vi "__replaceDupNames.vi"(10 "input names":string[](array[string])=["tt", "", "tt1", "tt0", "tt11", "", "Untitled1", "10t", "10t", "tt11", "Untitled", "tt001", "tt001", "tt2", "tt1.3", "tt1.3", "tt100", "tt100"]) -> (2 "output names":string[](array[string]))   [LabVIEW 2020]
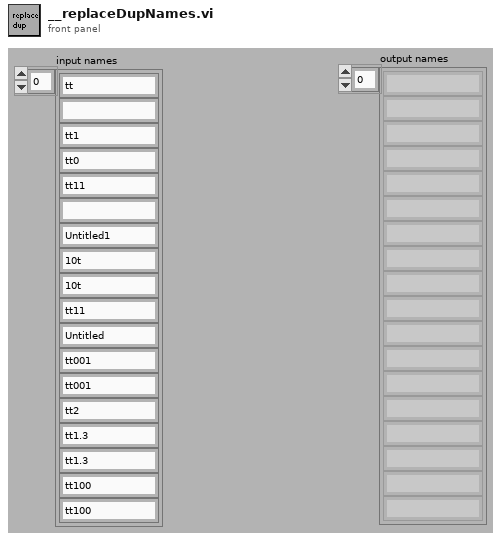
[diagram p1: front panel]
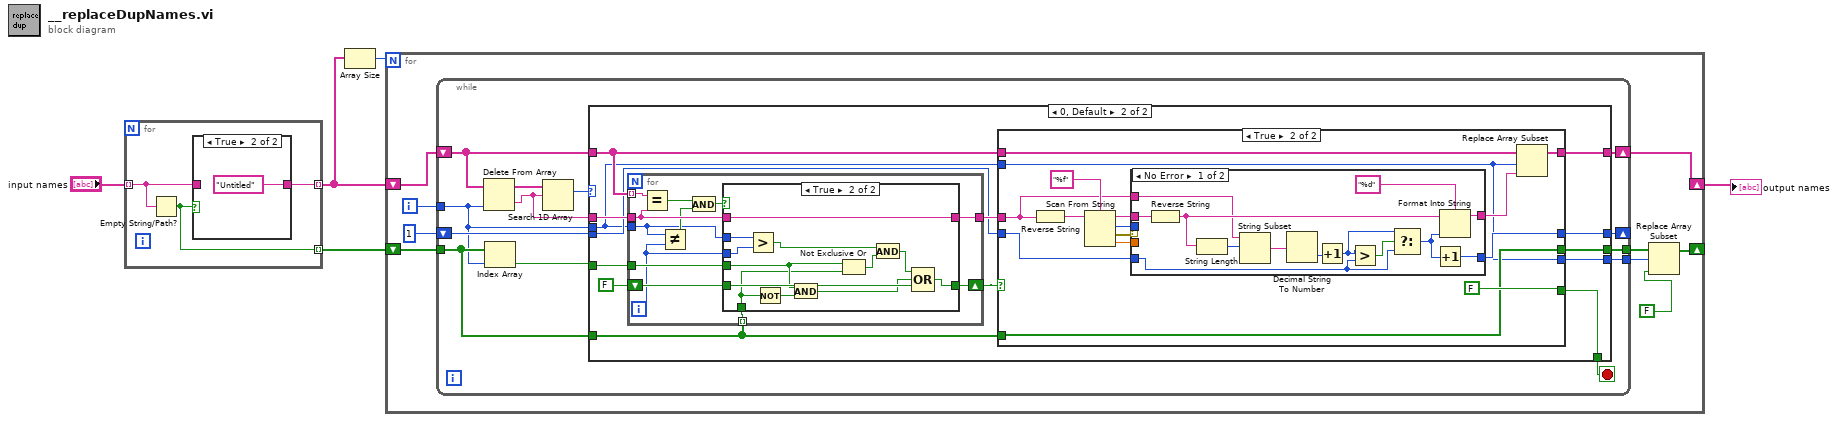
[diagram p0: block diagram]
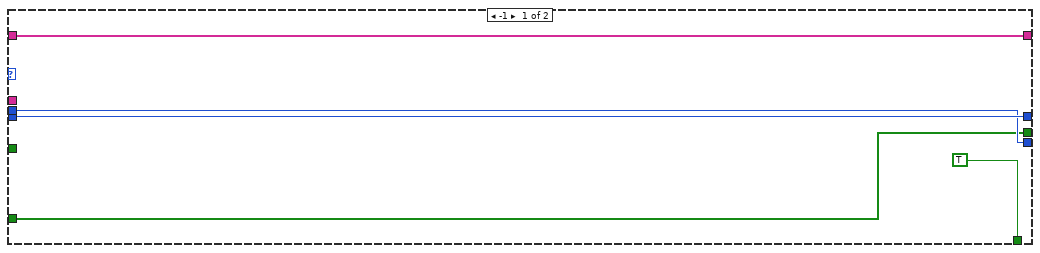
[diagram p2: hidden frame]
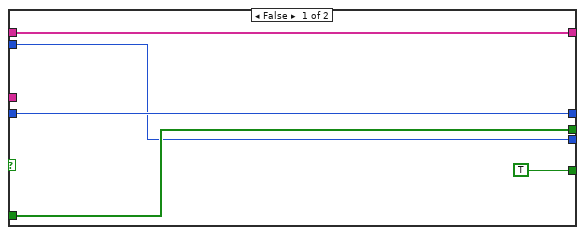
[diagram p4: hidden frame]
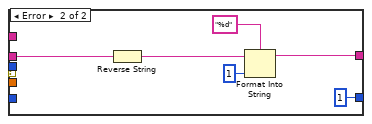
[diagram p5: hidden frame]
diagram:
  n1 = for {
    tunnel: "input names" -> [w8] mode=indexing
    tunnel: [w7] -> w3 mode=indexing
    tunnel: [w6] -> w2 mode=indexing
    n2 = Empty String/Path?(string/path=w8) -> (empty?=w6:bool)
    n3 = case shown="True" w6 {
      tunnel: w8 -> [w9 _]
      tunnel: [w9 "Untitled" ("Value")] -> w7
      frame False {
      }
      frame True {
      }
    }
  }
  n4 = Array Size(array=w3) -> (size(s)=w1:i32)
  n5 = for {
    N: w1 -> [_]
    shift-right: [w18] -> w4
    shift-left: w3 -> [w19]
    shift-right: [w13] -> _
    shift-left: w2 -> [w17]
    i -> [w15]
    n6 = while {
      tunnel: [w24] -> w14
      shift-right: [w31] -> w18
      shift-left: w19 -> [w28]
      tunnel: w17 -> [w22]
      shift-right: [w25] -> _
      shift-left: 1 -> [w29]
      tunnel: w15 -> [w21]
      tunnel: [w23] -> w11
      stop <- w32 stop-if-true
      n7 = Delete From Array(array=w28, index=w21) -> (deleted portion=w26:string, array with subset deleted=w27:string[])  [unwired: 1 in]
      n8 = Index Array(array=w22, index=w21) -> (element=w20:bool)
      n9 = Search 1D Array(1D array=w27, element=w26) -> (index of element=w30:i32)  [unwired: 1 out]
      n10 = case shown="0, Default" w30 {
        tunnel: [w33 w51] -> w24
        tunnel: w28 -> [w36 w46]
        tunnel: [TRUE ("new element/subarray") w48] -> w32
        tunnel: [w36 w50] -> w31
        tunnel: w26 -> [_ w45]
        tunnel: w29 -> [w35 w40]
        tunnel: [w35 w49] -> w25
        tunnel: w21 -> [w34 w38]
        tunnel: [w34 w47] -> w23
        tunnel: w22 -> [w33 w41]
        tunnel: w20 -> [_ w42]
        frame -1 {
        }
        frame 0, Default {
          n11 = for {
            tunnel: w46 -> [w63] mode=indexing
            tunnel: w45 -> [w62]
            tunnel: [w61] -> w44
            shift-right: [w59] -> w39
            shift-left: FALSE -> [w60]
            tunnel: w42 -> [w57]
            tunnel: w41 -> [w58] mode=indexing
            tunnel: w38 -> [w53]
            i -> [w52]
            n12 = Equal?(x=w63, y=w62) -> (x = y?=w56:bool)
            n13 = Not Equal?(x=w53, y=w52) -> (x != y?=w55:bool)
            n14 = And(x=w56, y=w55) -> (x .and. y?=w54:bool)
            n15 = case shown="True" w54 {
              tunnel: w62 -> [w65 w73]
              tunnel: [w65 w73] -> w61
              tunnel: w60 -> [w64 w76]
              tunnel: [w64 w77] -> w59
              tunnel: w58 -> [_ w69]
              tunnel: w57 -> [_ w70]
              tunnel: w53 -> [_ w72]
              tunnel: w52 -> [_ w71]
              frame False {
              }
              frame True {
                n16 = Greater?(x=w72, y=w71) -> (0:w67:bool)
                n17 = Not(x=w69) -> (.not. x?=w75:bool)
                n18 = And(x=w70, y=w75) -> (x .and. y?=w74:bool)
                n19 = Not Exclusive Or(1:w69, 2:w70) -> (0:w68:bool)
                n20 = And(x=w67, y=w68) -> (x .and. y?=w66:bool)
                n21 = Compound Arithmetic op=OR(w66, w74, w76) -> (w77:bool)
              }
            }
          }
          n22 = case shown="True" w39 {
            tunnel: [w80 w84] -> w51
            tunnel: w46 -> [w81 w97]
            tunnel: [w81 w89] -> w50
            tunnel: w41 -> [w80 w84]
            tunnel: w44 -> [_ w88]
            tunnel: w40 -> [w82 w85]
            tunnel: [w82 w87] -> w49
            tunnel: [TRUE ("new element/subarray") FALSE ("new element/subarray")] -> w48
            tunnel: w38 -> [w78 w83]
            tunnel: [w78 w83] -> w47
            frame False {
            }
            frame True {
              n23 = Reverse String(1:w88) -> (0:w90:string)
              n24 = Scan From String(format string="%f", input string=w90) -> (remaining string=w95:string, offset past scan=w91:u32, error out=w94:errorcluster, output 1=w92:dbl)  [unwired: 2 in, 1 out]
              n25 = case shown="No Error" w94 {
                tunnel: [w110 w116] -> w93
                tunnel: w95 -> [w107 w114]
                tunnel: w92 -> [_ _]
                tunnel: w91 -> [_ _]
                tunnel: w88 -> [w104 _]
                tunnel: w85 -> [w98 _]
                tunnel: [w103 1] -> w87
                frame No Error {
                  n26 = Reverse String(1:w107) -> (0:w105:string)
                  n27 = String Length(string=w105) -> (length=w106:i32)
                  n28 = String Subset(string=w104, offset (0)=w106) -> (substring=w108:string)  [unwired: 1 out]
                  n29 = Decimal String To Number(string=w108) -> (number=w102:i32)  [unwired: 3 out]
                  n30 = Increment(x=w102) -> (x+1=w99:i32)
                  n31 = Greater?(x=w99, y=w98) -> (0:w100:bool)
                  n32 = Select(t=w99, s=w100, f=w98) -> (s? t:f=w101:i32)
                  n33 = Increment(x=w101) -> (x+1=w103:i32)
                  n34 = Format Into String(format string="%d", initial string=w105, w101) -> (resulting string=w110:string)  [unwired: 1 in, 1 out]
                }
                frame Error {
                  n35 = Reverse String(1:w114) -> (0:w113:string)
                  n36 = Format Into String(format string="%d", initial string=w113, 1 ("input 1")) -> (resulting string=w116:string)  [unwired: 1 in, 1 out]
                }
              }
              n37 = Replace Array Subset(array=w97, new element=w93, index=w83) -> (w89:string[])
            }
          }
        }
      }
    }
    n38 = Replace Array Subset(array=w14, new element=FALSE ("new element/subarray"), index=w11) -> (w13:bool[])
  }
  "output names" <- w4
